vi "Write Light State.vi"(8 "error in":errorcluster, 10 "Light Mode":T1, 11 "Light Stack in":refnum<class "Light Stack.lvclass">) -> (0 "error out":errorcluster, 3 "Light Stack out":refnum<class "Light Stack.lvclass">)   [LabVIEW 2018, in "Light Stack.lvlib" / "Light Stack.lvclass"]
uses:
  Light Stack.lvclass
  Custom Controls/Light Mode.ctl
  Light Stack.lvclass/Light Stack.ctl
  Light Stack.lvlib
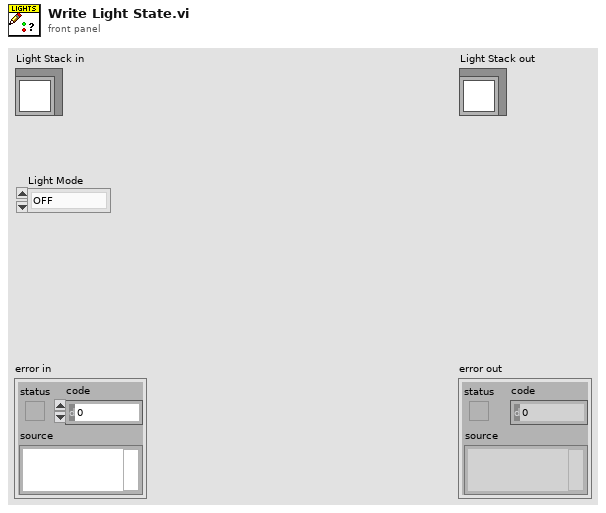
[diagram p1: front panel]
types:
  T1 = typedef "Light Stack.lvlib/Light Mode.ctl" = enum16{"OFF", "ON", "BLINK"}
  T2 = typedef "Light Stack.lvlib/Light Select.ctl" = enum16{"Red", "Amber", "Green", "Blue"}
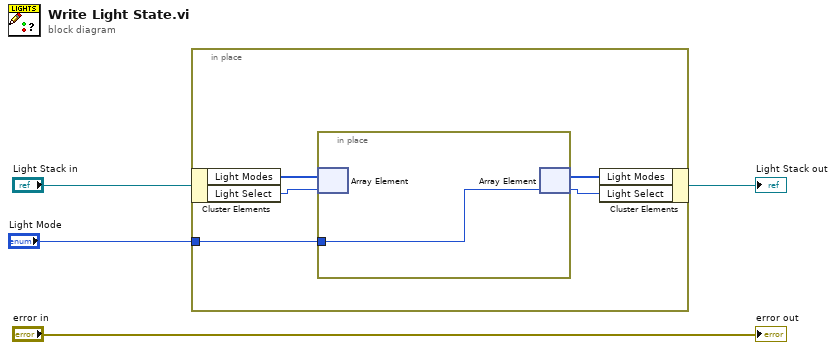
[diagram p0: block diagram]
diagram:
  n1 = in-place {
    in-place-border: "Light Mode" -> [w6]
    n2 = in-place-cluster #1("Light Stack in") -> ("Light Modes"=w9:T1[], "Light Select"=w7:T2)
    n3 = in-place {
      in-place-border: w6 -> [w10]
      n4 = in-place-array #2(w9, w7) -> ()  [unwired: 1 out]
      n5 = in-place-array #2(w10) -> (w8:T1[], w5:i32)
    }
    n6 = in-place-cluster #1("Light Modes"=w8, "Light Select"=w5) -> (→"Light Stack out":refnum<class "Light Stack.lvclass">)
  }
  "error out" <- "error in"
